vi "SetAnalogOutSourceSignal.vi"(8 "Error in":errorcluster, 9 "SourceSignal":refnum<k24>, 10 "OutputSignal":refnum<k24>, 11 "DevicesAndSignals":T1) -> (0 "Error out":errorcluster, 3 "DevicesAndSignals":T1)   [LabVIEW 2016]
doc: "Sets the source signal for an analog out signal to the given source.\n\nOutputSignal: Analog out signal to configure (has to be of type AnalogOutSignal).\nSourceSignal: Signal whose measurement values should be transformed into an output voltage at the physical connector of the given output signal (according to the output scaling settings of the output signal)."
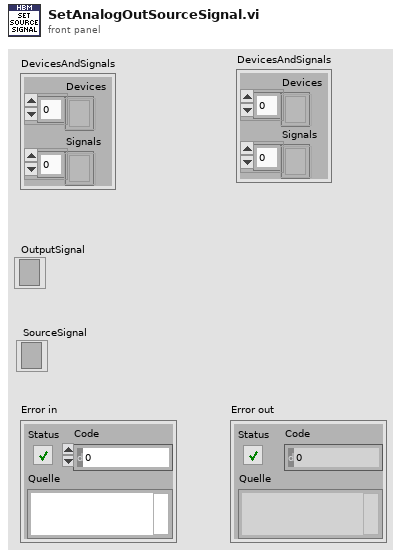
[diagram p1: front panel]
types:
  T1 = cluster{"Devices":refnum<k24>[], "Signals":refnum<k24>[]}
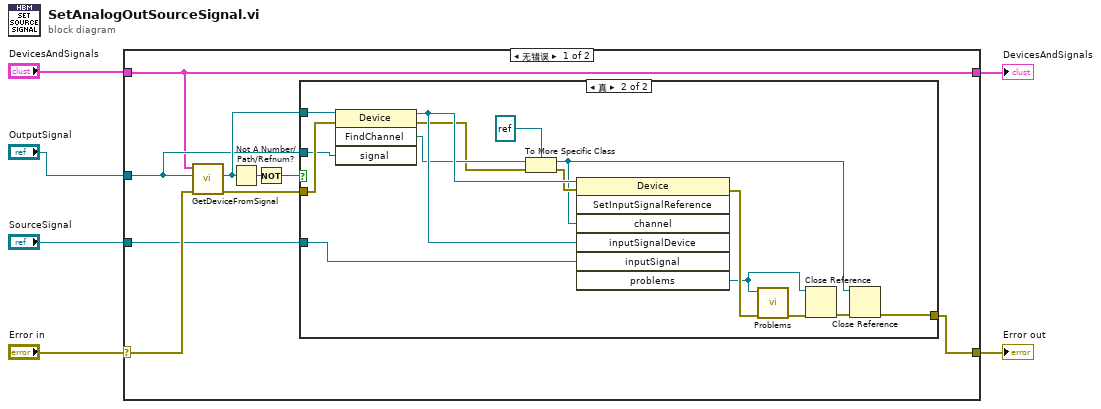
[diagram p0: block diagram]
diagram:
  n1 = case shown="无错误" "Error in" {
    selector: "Error in" -> [w15 w33]
    tunnel: [w8 w33] -> w5
    tunnel: "DevicesAndSignals" -> [w7 w32]
    tunnel: [w7 w32] -> w3
    tunnel: "OutputSignal" -> [w10 _]
    tunnel: "SourceSignal" -> [w9 _]
    frame No Error {
      n2 = call "GetDeviceFromSignal.vi"("Error in"=w15, "Signal"=w10, "DevicesAndSignals"=w7) -> ("Error out"=w11:errorcluster, "Device"=w12:refnum<k24>)  [unwired: 6 in, 1 out]
      n3 = Not A Number/Path/Refnum?(number/path/refnum=w12) -> (NaN/Path/Refnum?=w13:bool)
      n4 = Not(x=w13) -> (.not. x?=w14:bool)
      n5 = case shown="真" w14 {
        tunnel: w12 -> [_ w29]
        tunnel: w11 -> [w16 w31]
        tunnel: w10 -> [_ w30]
        tunnel: w9 -> [_ w27]
        tunnel: [w16 w17] -> w8
        frame False {
        }
        frame True {
          n6 = invoke on="Methodenknoten" class="Device" method="FindChannel"(reference=w29, error in=w31, "signal"=w30) -> (reference out=w28:refnum<k24>, error out=w23:errorcluster, "FindChannel"=w26:refnum<k24>)  [unwired: 1 in, 1 out]
          n7 = To More Specific Class(target class=refnum<k24> refnum (".NET (Referenz)"), reference=w26, error in=w23) -> (specific class reference=w18:refnum<k24>, error out=w25:errorcluster)
          n8 = invoke on="Methodenknoten" class="Device" method="SetInputSignalReference"(reference=w28, error in=w25, "channel"=w18, "inputSignalDevice"=w28, "inputSignal"=w27) -> (error out=w24:errorcluster, "problems"=w20:refnum<k24>)  [unwired: 2 in, 5 out]
          n9 = call "Problems.vi"("Error in"=w24, "Problems"=w20) -> ("Error out"=w21:errorcluster)  [unwired: 9 in]
          n10 = Close Reference(reference=w20, error in (no error)=w21) -> (error out=w19:errorcluster)
          n11 = Close Reference(reference=w18, error in (no error)=w19) -> (error out=w17:errorcluster)
        }
      }
    }
    frame Error {
    }
  }
  "Error out" <- w5
  "DevicesAndSignals" <- w3
